vi "Return Stamp Precheck.vi"(8 "error in (no error)":errorcluster, 10 "Slot Number":i32, 11 "GrabberTool Class in":refnum<class "GrabberTool Class.lvclass">) -> (0 "error out":errorcluster, 3 "GrabberTool Class out":refnum<class "GrabberTool Class.lvclass">)   [LabVIEW 2011, in "GrabberTool Class.lvclass"]
uses:
  GrabberTool Class.lvclass
  WorkTable Class/WorkTable Class.lvclass
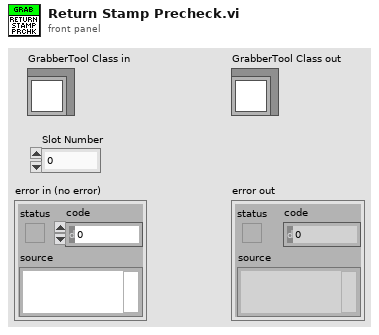
[diagram p1: front panel]
types:
  T1 = typedef "Worktable_Stamp.ctl" = cluster{"Stamp State":enum16{"Empty", "Populated", "Used"}, "Location/Orientation":T2, "Stamp Type":T3}
  T2 = typedef "Position_Orientation.ctl" = cluster{"Center":refnum<class "Vec3d Class.lvclass">, "Orientation":refnum<class "Orient3d Class.lvclass">}
  T3 = typedef "Stamp Type.ctl" = enum16{"Stamp 1", "Stamp 2", "Stamp 3", "Stamp 4"}
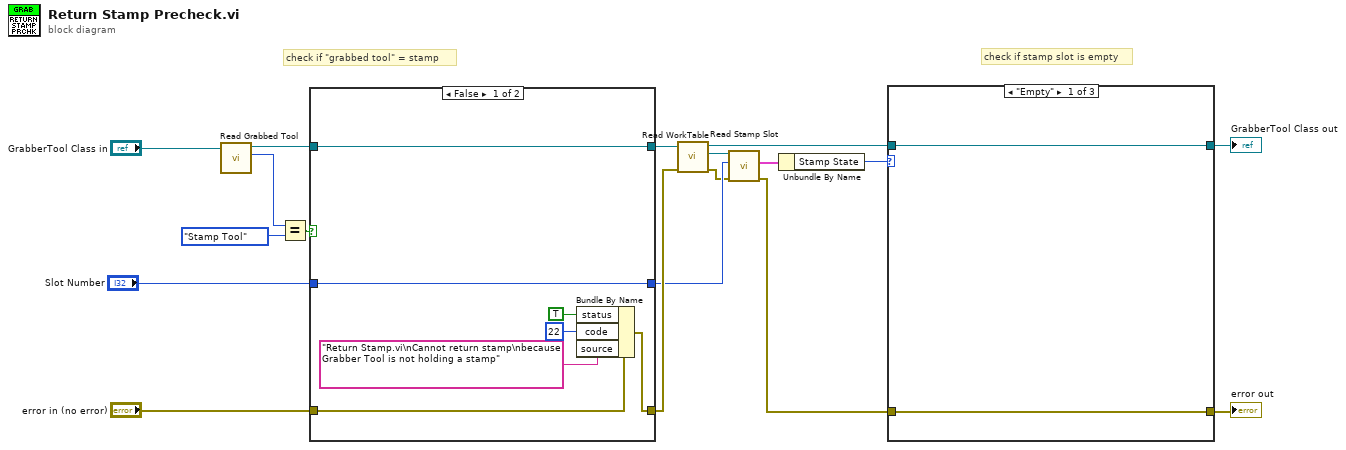
[diagram p0: block diagram]
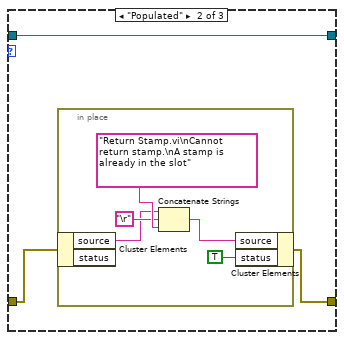
[diagram p2: hidden frame]
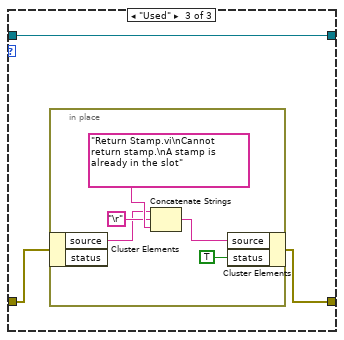
[diagram p3: hidden frame]
diagram:
  # "check if stamp slot is empty"
  # "check if \"grabbed tool\" = stamp"
  n1 = call "Read Grabbed Tool.vi"("GrabberTool Class in"="GrabberTool Class in") -> ("Grabbed Tool"=w12:enum16{"Weight Tool", "Stamp Tool", "Nothing"}, "GrabberTool Class out"=w11:refnum<class "GrabberTool Class.lvclass">)  [unwired: 8 in, 1 out]
  n2 = Equal?(x=w12, y=enum16{"Weight Tool", "Stamp Tool", "Nothing"}."Stamp Tool") -> (x = y?=w17:bool)
  n3 = case shown="False" w17 {
    tunnel: [w23 w27] -> w14
    tunnel: [w25 w28] -> w15
    tunnel: w11 -> [w25 w28]
    tunnel: "error in (no error)" -> [w24 w27]
    tunnel: "Slot Number" -> [w19 w26]
    tunnel: [w19 w26] -> w8
    frame False {
      n4 = Bundle By Name(cluster=w24, "status"=TRUE, "code"=22, "source"="Return Stamp.vi\nCannot return stamp\nbecause Grabber Tool is not holding a stamp") -> (w23:errorcluster)
    }
    frame True {
    }
  }
  n5 = call-dynamic "Read WorkTable.vi"("error in"=w14, "Gantry Class in"=w15) -> ("error out"=w3:errorcluster, "WorkTable Class.lvclass"=w9:refnum<class "WorkTable Class.lvclass">, "Gantry Class out"=w5:refnum<class "GrabberTool Class.lvclass">)  [unwired: 7 in]
  n6 = call "Read Stamp Slot.vi"("error in (no error)"=w3, "Stamp Slot"=w8, "WorkTable Class in"=w9) -> ("error out"=w2:errorcluster, "Stamp Slot"=w7:T1)  [unwired: 6 in, 1 out]
  n7 = Unbundle By Name(w7) -> ("Stamp State"=w6:enum16{"Empty", "Populated", "Used"})
  n8 = case shown="\"Empty\"" w6 {
    tunnel: w5 -> [w30 w33 w39]
    tunnel: [w30 w33 w39] -> w4
    tunnel: w2 -> [w29 w32 w41]
    tunnel: [w29 w31 w40] -> w1
    frame "Empty" {
    }
    frame "Populated" {
      n9 = in-place {
        n10 = in-place-cluster #1(w32) -> ("source"=w35:string)  [unwired: 1 out]
        n11 = Concatenate Strings(w35, "\r", "Return Stamp.vi\nCannot return stamp.\nA stamp is already in the slot" ("string")) -> (w36:string)
        n12 = in-place-cluster #1("source"=w36, "status"=TRUE) -> (w31:errorcluster)
      }
    }
    frame "Used" {
      n13 = in-place {
        n14 = in-place-cluster #2(w41) -> ("source"=w43:string)  [unwired: 1 out]
        n15 = Concatenate Strings(w43, "\r", "Return Stamp.vi\nCannot return stamp.\nA stamp is already in the slot" ("string")) -> (w44:string)
        n16 = in-place-cluster #2("source"=w44, "status"=TRUE) -> (w40:errorcluster)
      }
    }
  }
  "error out" <- w1
  "GrabberTool Class out" <- w4
